vi "SECoP-setAddFocus.vi"(8 "error in (no error)":errorcluster, 10 "key name":string, 11 "DLL path (in)":T1) -> (0 "error out":errorcluster, 3 "DLL path (out)":T1)   [LabVIEW 2023, in "SECoP.lvlib"]
doc: "Call <b>\"SECoP-setAddFocus.vi\"</b> to change the focus while SEC node creation. If your creation is not able to guarantee the order of \"SECoP-add*.vi\" functions, you could use this function. Normally you should not need this. Use a colon (':') separated name for selecting the current item. Selectable items are nodes, modules, command and parameters.\n\n<b>DLL path</b> input and output of cluster from \"SECoP-Initialize.vi\"\n<b>key name</b> name of key to point to (node, module, parameter or command)"
uses:
  SECoP.lvlib
  SECoP-libraries.ctl
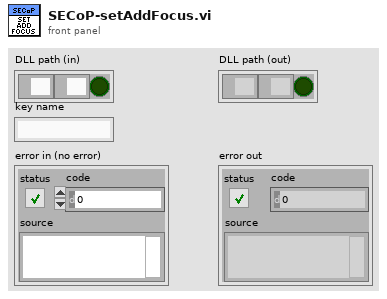
[diagram p1: front panel]
types:
  T1 = typedef "SECoP.lvlib/SECoP-libraries.ctl" = cluster{"serverDLL":path, "variantDLL":path, "cleanup_mode":bool}
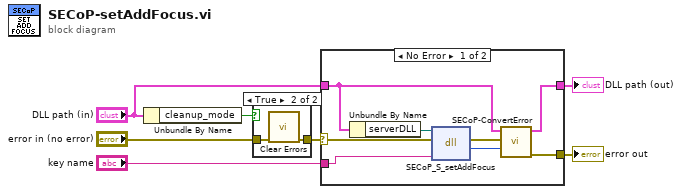
[diagram p0: block diagram]
diagram:
  n1 = Unbundle By Name("DLL path (in)") -> ("cleanup_mode"=w3:bool)
  n2 = case shown="True" w3 {
    tunnel: "error in (no error)" -> [w8 w10]
    tunnel: [w8 w9] -> w1
    frame False {
    }
    frame True {
      n3 = call <vilib>:"Clear Errors.vi"("error in (no error)"=w10) -> ("error out"=w9:errorcluster)  [unwired: 5 in, 1 out]
    }
  }
  n4 = case shown="No Error" w1 {
    selector: w1 -> [w16 w19]
    tunnel: "DLL path (in)" -> [w12 w20]
    tunnel: [w17 w20] -> w6
    tunnel: [w18 w19] -> w5
    tunnel: "key name" -> [w13 _]
    frame No Error {
      n5 = Unbundle By Name(w12) -> ("serverDLL"=w11:path)
      n6 = dll-call lib="Z:/Praktische Aufgaben/SECoP-LabVIEW2015/32bit/SECoP32.dll" fn="SECoP_S_setAddFocus"(path in=w11, error in=w16, "name(Key)"=w13) -> (error out=w15:errorcluster, "return type"=w14:i32)  [unwired: 2 in, 1 out]
      n7 = call "SECoP-ConvertError.vi"("return code"=w14, "error in (no error)"=w15, "DLL path (in)"=w12) -> ("error out"=w18:errorcluster, "DLL path (out)"=w17:T1)  [unwired: 7 in]
    }
    frame Error {
    }
  }
  "DLL path (out)" <- w6
  "error out" <- w5
